vi "Data Viewer.vi"() -> ()   [LabVIEW 2016]
uses:
  Libraries/File/Controls/Data Viewer Entry.ctl
  Libraries/File/Controls/Channel name entry.ctl
  Libraries/File/Controls/Data reduction.ctl
panel:
  in  "Relative time":bool
  out "Dy":dbl format="%#_4p"
  out "1/Dx":dbl format="%#_4p"
  out "Dx":dbl format="%#_4p"
  in  "Decimation method":T1(ring)=enum."Min-Max"
  in  "Max points (-1:all)":i32=1000000 format="%.0p"
  in  "Clip time":bool
  in  "Time interval":cluster{dbl, dbl}(slide)={0.1, -0.01} scale=-0.01..0.1 scale format="%#_6p"
  in  "Clear all":bool
  in  "stop":bool
  out "XY Graph":cluster{dbl[], dbl[]}[](graph)
  in  "Group name":string="Untitled"
  in  "Data files":T2[](array[typedef])
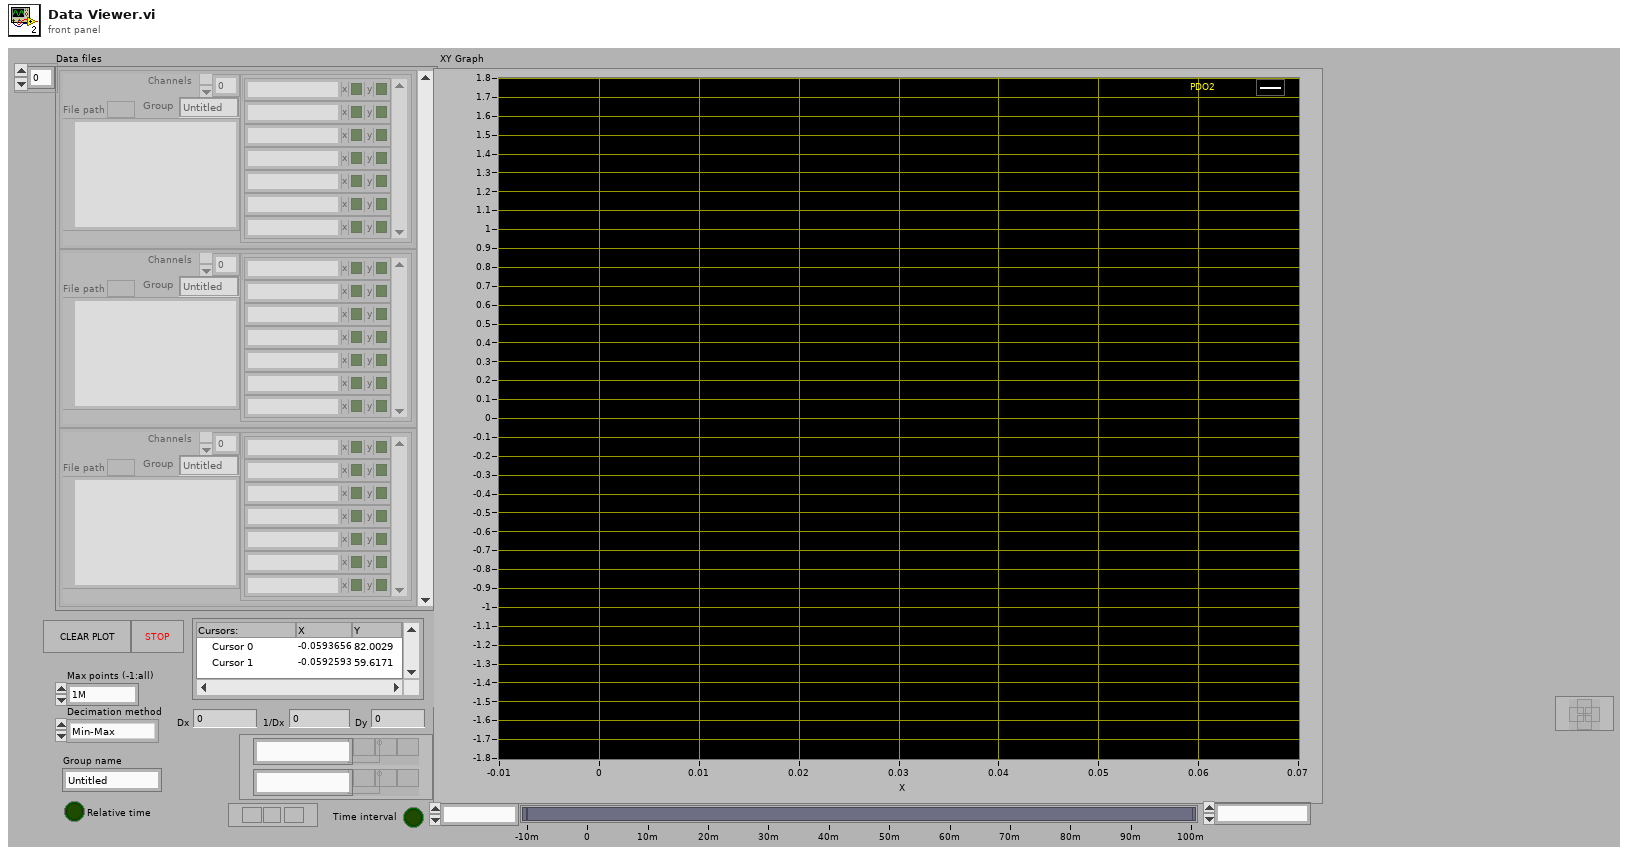
[diagram p1: front panel]
types:
  T1 = enum16{"coerce", "linear", "spline", "Min-Max", "Average"}
  T2 = typedef "Data Viewer Entry.ctl" = cluster{"File path":path, "Channels":T3[], "Group":string}
  T3 = typedef "Channel name entry.ctl" = cluster{"Name":string, "x":bool, "y":bool}
  T4 = typedef "Data reduction.ctl" = cluster{"Clip time":bool, "Tiime 0":dbl, "Time 1":dbl, "Maximum data points":i32, "Decimation method":enum16{"coerce", "linear", "spline", "Min-Max", "Average"}}
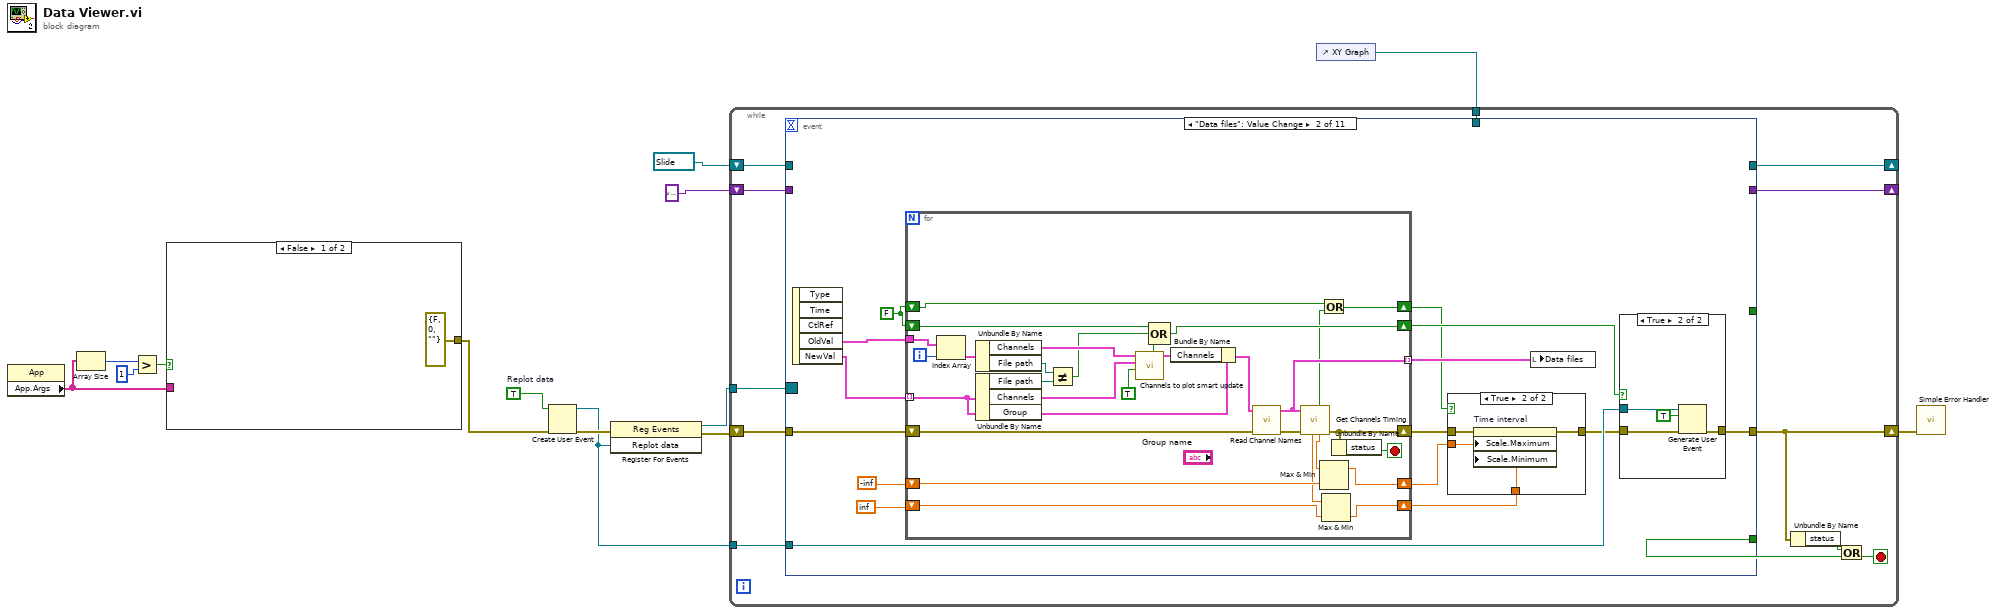
[diagram p0: block diagram]
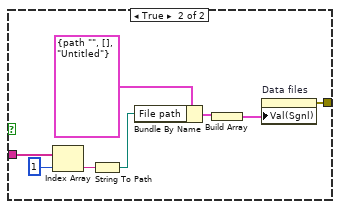
[diagram p2: hidden frame]
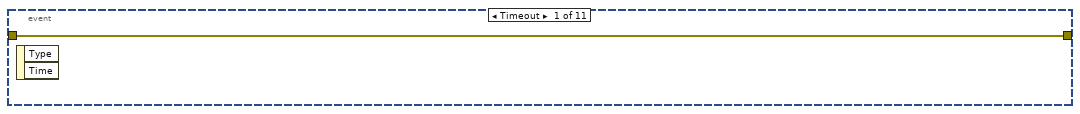
[diagram p3: hidden frame]
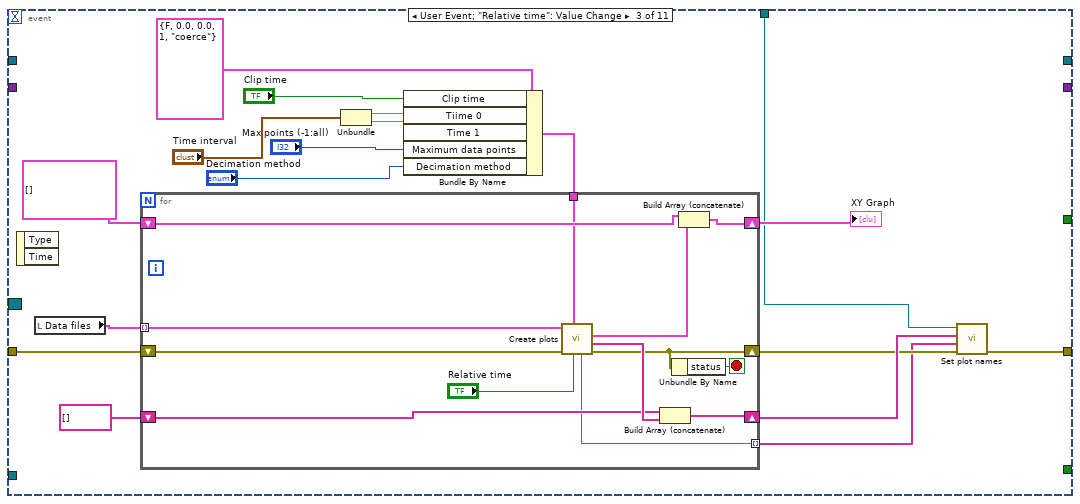
[diagram p6: hidden frame]
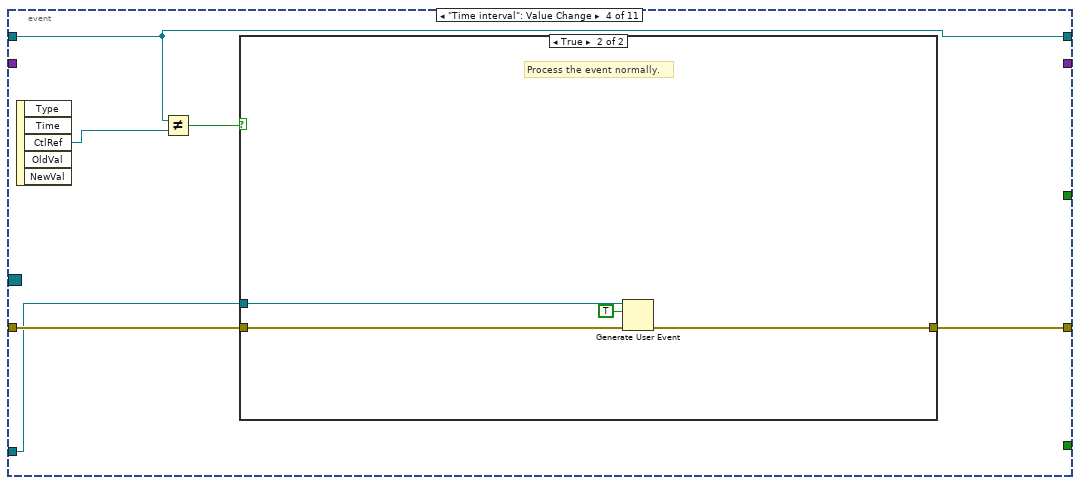
[diagram p7: hidden frame]
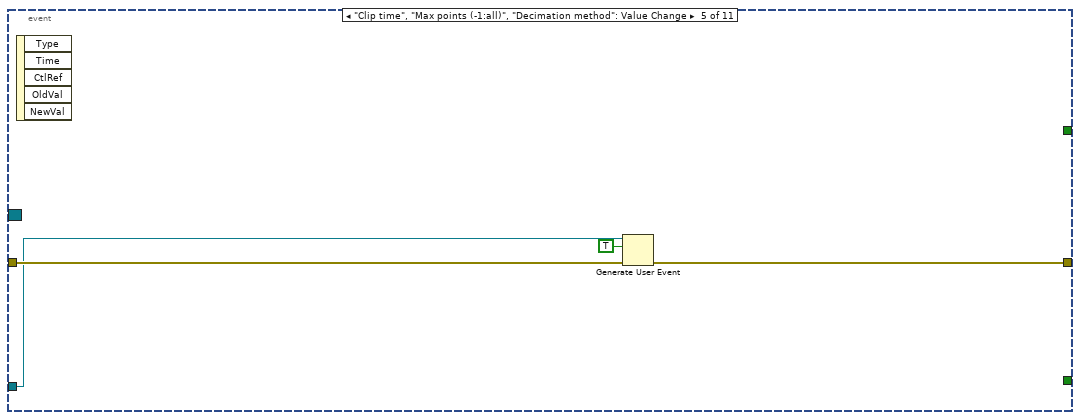
[diagram p9: hidden frame]
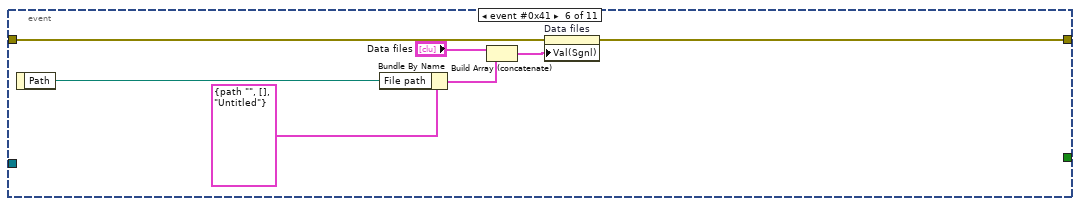
[diagram p10: hidden frame]
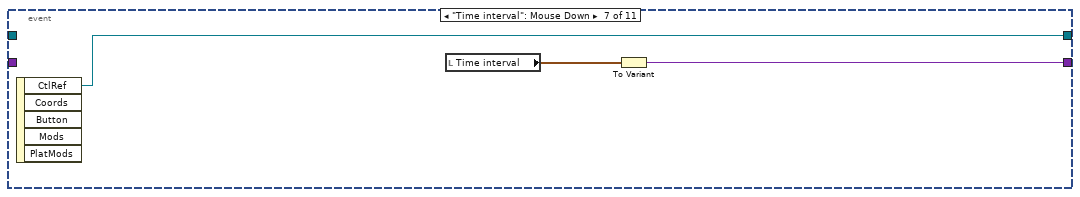
[diagram p11: hidden frame]
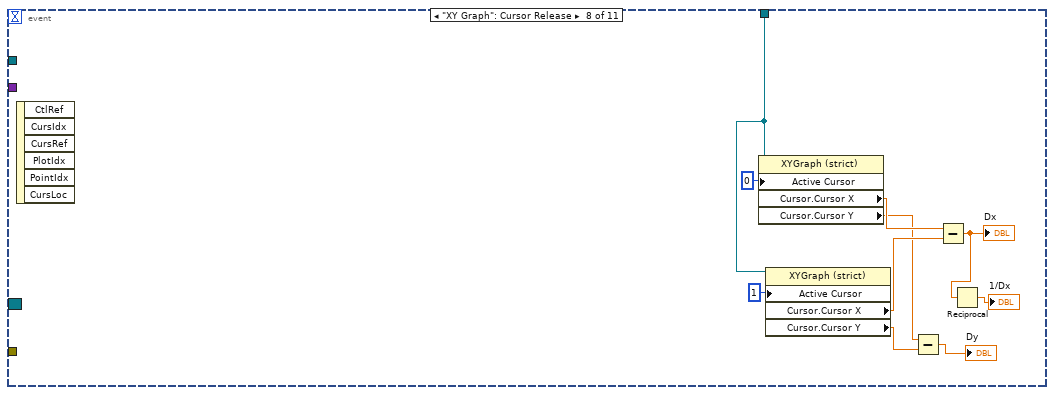
[diagram p12: hidden frame]
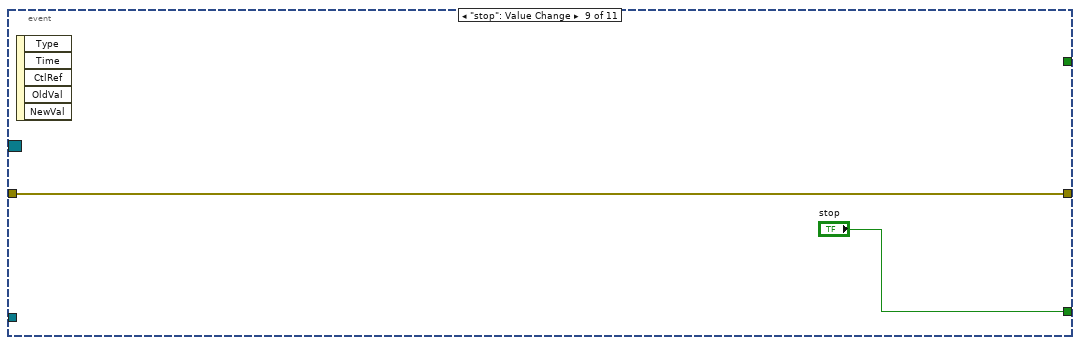
[diagram p13: hidden frame]
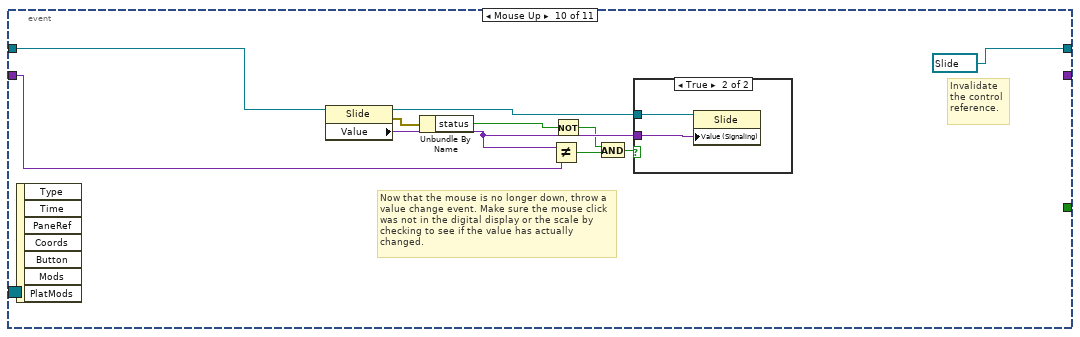
[diagram p14: hidden frame]
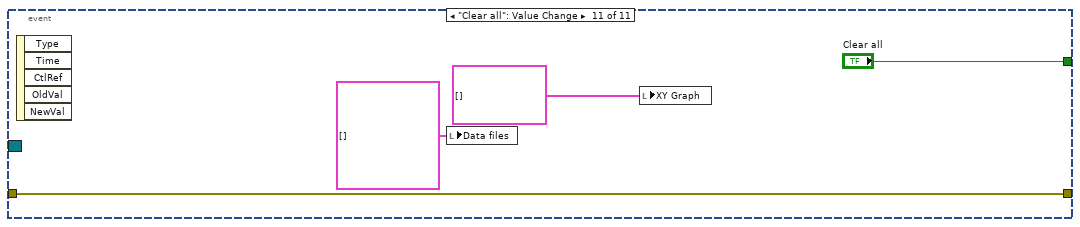
[diagram p16: hidden frame]
diagram:
  w9 = TRUE  # Replot data
  n1 = property class="App"() -> ("App.Args"=w13:string[])  [unwired: 2 in, 2 out]
  n2 = Array Size(array=w13) -> (size(s)=w12:i32)
  n3 = Greater?(x=w12, y=1) -> (0:w10:bool)
  n4 = case shown="False" w10 {
    tunnel: w13 -> [_ w23]
    tunnel: [errorcluster {"status"=FALSE, "code"=0, "source"=""} ("error out") w16] -> w7
    frame False {
    }
    frame True {
      n5 = Index Array(array=w23, index=1) -> (element=w21:string)
      n6 = String To Path(string=w21) -> (path=w19:path)
      n7 = Bundle By Name(cluster=T2 {"File path"=path "", "Channels"=[], "Group"="Untitled"} ("Cluster"), "File path"=w19) -> (w18:T2)
      n8 = Build Array(w18) -> (w17:T2[])
      n9 = property on="Data files" class="Arr (strict)"("Val(Sgnl)"=w17) -> (error out=w16:errorcluster)  [unwired: 2 in, 1 out]
    }
  }
  n10 = Create User Event(user event datatype=w9, error in=w7) -> (user event=w4:refnum<user-event>, error out=w8:errorcluster)
  n11 = register-events(error in=w8, w4) -> (reference out=w5:refnum<event-registration>, error out=w6:errorcluster)  [unwired: 1 in]
  n12 = control-ref of="XY Graph"() -> (w1:refnum<vi>)
  n13 = while {
    shift-right: [w31] -> w14
    shift-left: w6 -> [w35]
    tunnel: w5 -> [w30]
    tunnel: w4 -> [w29]
    shift-right: [w25] -> _
    shift-left: refnum<vi> refnum ("CtlRef") -> [w28]
    shift-right: [w26] -> _
    shift-left: variant ("Variant") -> [w27]
    tunnel: w1 -> [w24]
    stop <- w33 stop-if-true
    n14 = event shown="[1] \"Data files\": Value Change" {
      selector: w30 -> [_ _ _ _ _ _ _ _ _ _ _]
      dyn-events: _ -> [_ _ _ _ _ _ _ _ _ _ _]
      timeout: _ -> [_ _ _ _ _ _ _ _ _ _ _]
      tunnel: w35 -> [w36 w50 w108 w124 w136 w138 _ _ w158 _ w173]
      tunnel: [w36 w47 w105 w123 w135 w137 _ _ w158 _ w173] -> w31
      tunnel: [_ _ _ _ _ _ _ _ "stop" _ _] -> w34
      tunnel: [_ _ _ _ _ _ _ _ _ _ "Clear all"] -> _
      tunnel: w29 -> [_ w48 _ w122 w134 _ _ _ _ _ _]
      tunnel: w28 -> [_ _ _ w125 _ _ _ _ _ w161 _]
      tunnel: w27 -> [_ _ _ _ _ _ _ _ _ w160 _]
      tunnel: [_ _ _ _ _ _ w145 _ _ _ _] -> w26
      tunnel: [_ _ _ w125 _ _ w144 _ _ refnum<vi> refnum ("CtlRef") _] -> w25
      tunnel: w24 -> [_ _ w91 _ _ _ _ w155 _ _ _]
      event Timeout {
        n15 = event-data() -> ()  [unwired: 1 in, 2 out]
      }
      event "Data files": Value Change {
        w38 = FALSE
        n16 = event-data() -> ("OldVal"=w49:T2[], "NewVal"=w51:T2[])  [unwired: 1 in, 3 out]
        n17 = for {
          tunnel: w51 -> [w83] mode=indexing
          shift-right: [w74] -> w42
          shift-left: w50 -> [w84]
          tunnel: w49 -> [w88]
          tunnel: [w76] -> w45 mode=indexing
          shift-right: [w77] -> w46
          shift-left: w38 -> [w78]
          shift-right: [w71] -> w40
          shift-left: -inf -> [w72]
          shift-right: [w70] -> w39
          shift-left: inf -> [w68]
          shift-right: [w65] -> w37
          shift-left: w38 -> [w67]
          i -> [w87]
          stop <- w90 stop-if-true
          n18 = Index Array(array=w88, index=w87) -> (element=w86:T2)
          n19 = Unbundle By Name(w86) -> ("Channels"=w85:T3[], "File path"=w64:path)
          n20 = Unbundle By Name(w83) -> ("File path"=w63:path, "Channels"=w89:T3[])  [unwired: 1 out]
          n21 = Not Equal?(x=w64, y=w63) -> (x != y?=w62:bool)
          n22 = call "Channels to plot smart update.vi"("Disable y for 1st channel"=TRUE, "Channels to plot new value"=w89, "Channels to plot old value"=w85) -> ("Channels to plot out"=w82:T3[], "Replot?"=w79:bool)  [unwired: 1 in, 6 out]
          n23 = Compound Arithmetic op=OR(w78, w62, w79) -> (w77:bool)
          n24 = Bundle By Name(cluster=w83, "Channels"=w82) -> (w81:T2)
          n25 = call "Read Channel Names.vi"("error in"=w84, "Data record"=w81) -> ("error out"=w75:errorcluster, "Data record out"=w76:T2)  [unwired: 8 in]
          n26 = call "Get Channels Timing.vi"("error in (no error)"=w75, "Data file"=w76) -> ("error out"=w74:errorcluster, "Latest finish"=w73:dbl, "Plots exist"=w66:bool, "Earliest start"=w69:dbl)  [unwired: 5 in, 1 out]
          n27 = Or(x=w67, y=w66) -> (x .or. y?=w65:bool)
          n28 = Max & Min(x=w73, y=w72) -> (max(x,y)=w71:dbl)  [unwired: 1 out]
          n29 = Max & Min(x=w69, y=w68) -> (min(x,y)=w70:dbl)  [unwired: 1 out]
          n30 = Unbundle By Name(w74) -> ("status"=w90:bool)
        }
        n31 = case shown="True" w37 {
          tunnel: w42 -> [w52 w56]
          tunnel: [w52 w55] -> w41
          tunnel: w40 -> [_ w54]
          tunnel: w39 -> [_ w53]
          frame False {
          }
          frame True {
            n32 = property on="Time interval" class="Slide (strict)"(error in=w56, "Scale.Maximum"=w54, "Scale.Minimum"=w53) -> (error out=w55:errorcluster)  [unwired: 1 in, 1 out]
          }
        }
        n33 = local write "Data files"(w45) -> ()
        n34 = case shown="True" w46 {
          tunnel: w48 -> [_ w61]
          tunnel: w41 -> [w57 w60]
          tunnel: [w57 w59] -> w47
          frame False {
          }
          frame True {
            n35 = Generate User Event(user event=w61, event data cluster=TRUE ("event data"), error in=w60) -> (error out=w59:errorcluster)  [unwired: 1 in, 1 out]
          }
        }
      }
      event User Event; "Relative time": Value Change {
        n36 = event-data() -> ()  [unwired: 1 in, 2 out]
        n37 = local read "Data files"() -> (w101:T2[])
        n38 = Unbundle("Time interval") -> (w96:dbl, w95:dbl)
        n39 = Bundle By Name(cluster=T4 {"Clip time"=FALSE, "Tiime 0"=0.0, "Time 1"=0.0, "Maximum data points"=1, "Decimation method"=enum."coerce"} ("Data reduction"), "Clip time"="Clip time", "Tiime 0"=w96, "Time 1"=w95, "Maximum data points"="Max points (-1:all)", "Decimation method"="Decimation method") -> (w94:T4)
        n40 = for {
          shift-right: [w117] -> w104
          shift-left: w108 -> [w112]
          shift-right: [w119] -> w106
          shift-left: string[] [] -> [w118]
          shift-right: [w115] -> w100
          shift-left: cluster{sgl[], sgl[]}[] [] -> [w114]
          tunnel: [w113] -> w102 mode=indexing
          tunnel: w101 -> [w109] mode=indexing
          tunnel: w94 -> [w111]
          stop <- w121 stop-if-true
          n41 = call "Create plots.vi"("Relative time"="Relative time", "Data reduction"=w111, "error in (no error)"=w112, "Data record"=w109) -> ("error out"=w117:errorcluster, "Y names"=w120:string[], "Plots"=w116:cluster{dbl[], dbl[]}[], "X-axis name"=w113:string)  [unwired: 3 in, 1 out]
          n42 = Build Array (concatenate)(w118, w120) -> (w119:string[])
          n43 = Unbundle By Name(w117) -> ("status"=w121:bool)
          n44 = Build Array (concatenate)(w114, w116) -> (w115:cluster{dbl[], dbl[]}[])
        }
        "XY Graph" <- w100
        n45 = call "Set plot names.vi"("error in"=w104, "X-axis names"=w102, "Plot names"=w106, "XYGraph Refnum"=w91) -> ("error out"=w105:errorcluster)  [unwired: 6 in, 1 out]
      }
      event "Time interval": Value Change {
        n46 = event-data() -> ("CtlRef"=w127:refnum<vi>)  [unwired: 1 in, 4 out]
        n47 = Not Equal?(x=w125, y=w127) -> (x != y?=w126:bool)
        n48 = case shown="True" w126 {
          tunnel: w124 -> [w128 w131]
          tunnel: [w128 w130] -> w123
          tunnel: w122 -> [_ w129]
          frame False {
            # "Value changed, but the mouse button is still down, so disregard the event."
          }
          frame True {
            # "Process the event normally."
            n49 = Generate User Event(user event=w129, event data cluster=TRUE ("event data"), error in=w131) -> (error out=w130:errorcluster)  [unwired: 1 in, 1 out]
          }
        }
      }
      event "Clip time", "Max points (-1:all)", "Decimation method": Value Change {
        n50 = event-data() -> ()  [unwired: 1 in, 5 out]
        n51 = Generate User Event(user event=w134, event data cluster=TRUE ("event data"), error in=w136) -> (error out=w135:errorcluster)  [unwired: 1 in, 1 out]
      }
      event event #0x41 {
        n52 = event-data() -> ("Path"=w141:path)  [unwired: 1 in]
        n53 = Bundle By Name(cluster=T2 {"File path"=path "", "Channels"=[], "Group"="Untitled"} ("Cluster"), "File path"=w141) -> (w143:T2)
        n54 = Build Array (concatenate)("Data files", w143) -> (w139:T2[])
        n55 = property on="Data files" class="Arr (strict)"(error in=w138, "Val(Sgnl)"=w139) -> (error out=w137:errorcluster)  [unwired: 1 in, 1 out]
      }
      event "Time interval": Mouse Down {
        n56 = event-data() -> ("CtlRef"=w144:refnum<vi>)  [unwired: 1 in, 4 out]
        n57 = local read "Time interval"() -> (w146:cluster{dbl, dbl})
        n58 = To Variant(anything=w146) -> (Variant=w145:variant)
      }
      event "XY Graph": Cursor Release {
        n59 = event-data() -> ()  [unwired: 1 in, 6 out]
        n60 = property class="XYGraph (strict)"(reference=w155, "Active Cursor"=0 ("Cursor.Cursor Index")) -> ("Cursor.Cursor X"=w153:dbl, "Cursor.Cursor Y"=w149:dbl)  [unwired: 1 in, 2 out]
        n61 = property class="XYGraph (strict)"(reference=w155, "Active Cursor"=1 ("Cursor.Cursor Index")) -> ("Cursor.Cursor X"=w152:dbl, "Cursor.Cursor Y"=w148:dbl)  [unwired: 1 in, 2 out]
        n62 = Subtract(x=w149, y=w148) -> (x-y=→"Dy":dbl)
        n63 = Subtract(x=w153, y=w152) -> (x-y=w150:dbl)
        "Dx" <- w150
        n64 = Reciprocal(x=w150) -> (1/x=→"1/Dx":dbl)
      }
      event "stop": Value Change {
        n65 = event-data() -> ()  [unwired: 1 in, 5 out]
      }
      event Mouse Up {
        # "Invalidate\nthe control\nreference."
        # "Now that the mouse is no longer down, throw a value change event. Make sure the mouse click was not in the digital display or the scale by checking to see if the value has actually changed."
        n66 = event-data() -> ()  [unwired: 1 in, 7 out]
        n67 = property class="Slide"(reference=w161) -> (reference out=w168:refnum<vi>, error out=w167:errorcluster, "Value"=w166:variant)  [unwired: 1 in]
        n68 = Unbundle By Name(w167) -> ("status"=w164:bool)
        n69 = Not Equal?(x=w166, y=w160) -> (x != y?=w165:bool)
        n70 = Not(x=w164) -> (.not. x?=w162:bool)
        n71 = And(x=w162, y=w165) -> (x .and. y?=w163:bool)
        n72 = case shown="True" w163 {
          tunnel: w166 -> [_ w170]
          tunnel: w168 -> [_ w169]
          frame False {
          }
          frame True {
            n73 = property class="Slide"(reference=w169, "Value (Signaling)"=w170) -> ()  [unwired: 1 in, 2 out]
          }
        }
      }
      event "Clear all": Value Change {
        n74 = event-data() -> ()  [unwired: 1 in, 5 out]
        n75 = local write "Data files"(T2[] [] ("Data files")) -> ()
        n76 = local write "XY Graph"(cluster{dbl[], dbl[]}[] [] ("XY Graph")) -> ()
      }
    }
    n77 = Unbundle By Name(w31) -> ("status"=w32:bool)
    n78 = Or(x=w32, y=w34) -> (x .or. y?=w33:bool)
  }
  n79 = call <vilib>:"Simple Error Handler.vi"("error in (no error)"=w14) -> ()  [unwired: 4 in, 5 out]
